vi "Calculate panel colours.vi"(3 "Cp_min clamp (for 3D rendering)":sgl=-4.0 format="%#_6f", 4 "Cp_max clamp (for 3D rendering)":sgl=1.0 format="%#_6f", 5 "Cp":sgl[](array[numeric])) -> (0 "Cp_min":sgl, 1 "Cp_max":sgl, 2 "Panel colours":T1[](array[typedef]))   [LabVIEW 2017]
uses:
  <vilib>/Utility/miscctls.llb/LVRGBAColorTypeDef.ctl
panel:
  # "PN 26/10/17"
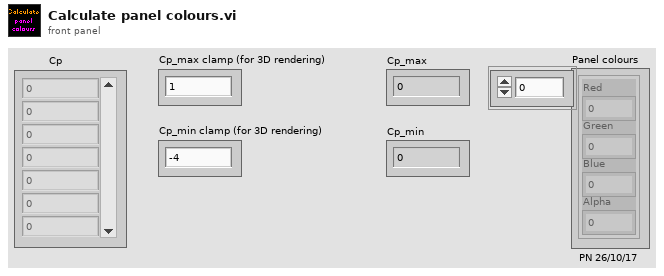
[diagram p1: front panel]
types:
  T1 = typedef "LVRGBAColorTypeDef.ctl" = cluster{"Red":sgl, "Green":sgl, "Blue":sgl, "Alpha":sgl}
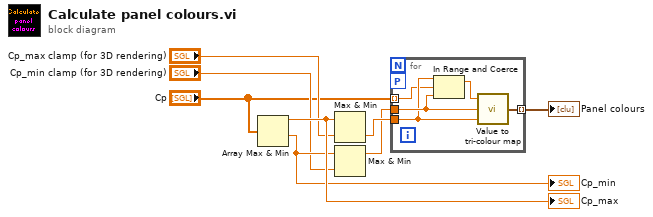
[diagram p0: block diagram]
diagram:
  n1 = Array Max & Min(array="Cp") -> (max value=w8:sgl, min value=w6:sgl)  [unwired: 2 out]
  "Cp_min" <- w6
  "Cp_max" <- w8
  n2 = Max & Min(x=w8, y="Cp_max clamp (for 3D rendering)") -> (min(x,y)=w7:sgl)  [unwired: 1 out]
  n3 = Max & Min(x=w6, y="Cp_min clamp (for 3D rendering)") -> (max(x,y)=w5:sgl)  [unwired: 1 out]
  n4 = for {
    tunnel: "Cp" -> [w10] mode=indexing
    workers-P: _ -> [_]
    tunnel: w7 -> [w11]
    tunnel: w5 -> [w12]
    tunnel: [w13] -> w2 mode=indexing
    n5 = In Range and Coerce(upper limit=w11, x=w10, lower limit=w12) -> (coerced(x)=w9:sgl)  [unwired: 1 out]
    n6 = call "Value to tri-colour map.vi"("Vmax"=w11, "Vmin"=w12, "V"=w9) -> ("Colour out"=w13:T1)
  }
  "Panel colours" <- w2
